vi "CheckSizeAndRefreshFile.vi"(8 "error in (no error)":errorcluster, 10 "MaxFileSize":i32, 11 "LogfileRef In":refnum<file>) -> (0 "error out":errorcluster, 3 "LogfileRef Out":refnum<file>)   [LabVIEW 2016, in "Log4Lv.lvlib"]
doc: "Use this template to build a VI to use as a subVI."
uses:
  Log4Lv.lvlib
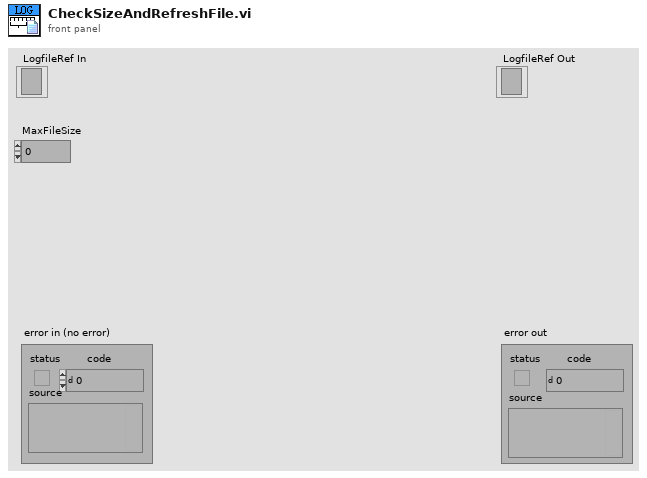
[diagram p1: front panel]
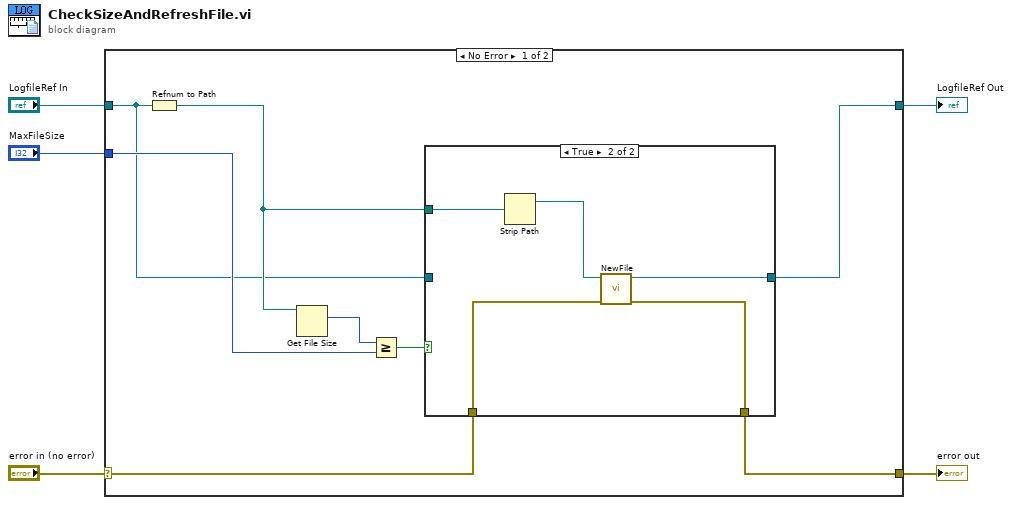
[diagram p0: block diagram]
diagram:
  n1 = case shown="No Error" "error in (no error)" {
    selector: "error in (no error)" -> [w7 w22]
    tunnel: [w6 w22] -> w4
    tunnel: "LogfileRef In" -> [w8 w21]
    tunnel: "MaxFileSize" -> [w12 _]
    tunnel: [w9 w21] -> w1
    frame No Error {
      n2 = Refnum to Path(1:w8) -> (0:w10:path)
      n3 = Get File Size(file=w10) -> (size (in bytes)=w13:i64)  [unwired: 1 in, 2 out]
      n4 = Greater Or Equal?(x=w13, y=w12) -> (x >= y?=w11:bool)
      n5 = case shown="True" w11 {
        tunnel: w10 -> [_ w20]
        tunnel: [w15 w17] -> w9
        tunnel: w8 -> [w15 _]
        tunnel: w7 -> [w14 w19]
        tunnel: [w14 w18] -> w6
        frame False {
        }
        frame True {
          n6 = Strip Path(path=w20) -> (stripped path=w16:path)  [unwired: 1 out]
          n7 = call "NewFile.vi"("error in (no error)"=w19, "LogFolder"=w16) -> ("error out"=w18:errorcluster, "LogfileRef Out"=w17:refnum<file>)  [unwired: 8 in]
        }
      }
    }
    frame Error {
    }
  }
  "error out" <- w4
  "LogfileRef Out" <- w1
